vi "Peaks & Baseline.vi"(0 "Y data":dbl[](array[numeric]) format="%.2f", 1 "X interval (1.0)":dbl=1.0 format="%.2f", 2 "tuning parameters\n(0:auto-calc)":T1 {"peak threshold" min=0.0 format="%.2f"; "max noise" min=0.0 format="%.2f"}, 3 "iteration (0:init)":i32) -> (6 "baseline":T2 {"Y" format="%.2f"; "X" format="%.2f"}, 7 "X,Y data":T2 {"Y" format="%.2f"; "X" format="%.2f"}, 8 "peak starts":T2 {"Y" format="%.2f"; "X" format="%.2f"}, 9 "peak maxima":T2 {"Y" format="%.2f"; "X" format="%.2f"}, 10 "peak ends":T2 {"Y" format="%.2f"; "X" format="%.2f"})   [LabVIEW 2012]
doc: "The Peaks & Baseline VI finds the start, maximum, and end of each peak in a signal, and a linear baseline. This VI can process all the data at once (post-processing), or it can process the data in segments (\"on-line\" or \"real-time\" processing). It keeps state information from one call to the next by using uninitialized shift registers, so it can process segmented data seamlessly. Iteration must be set to zero for the first call so the state information can be initialized.\n\nUse the help window to read the descriptions of the individual controls for more information about this VI's inputs and outputs."
uses:
  XY Plot.ctl
  Tuning.ctl
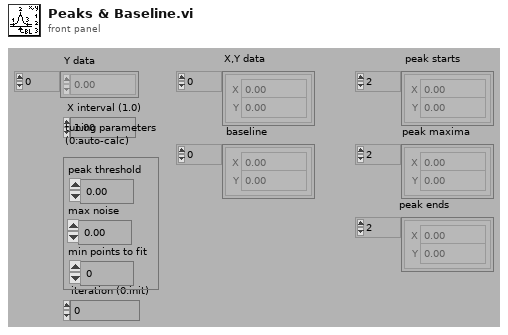
[diagram p1: front panel]
types:
  T1 = typedef "Tuning.ctl" = cluster{"max noise":dbl, "min points to fit":i32, "peak threshold":dbl}
  T2 = typedef "XY Plot.ctl" = cluster{"X":dbl, "Y":dbl}[]
  T3 = enum16{"initialize", "on baseline", "peak going up", "peak going down"}
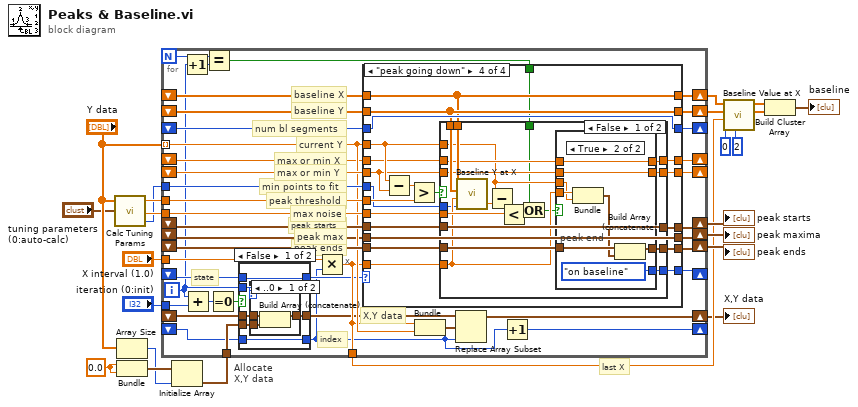
[diagram p0: block diagram]
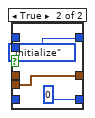
[diagram p3: hidden frame]
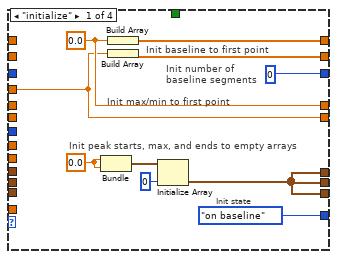
[diagram p4: hidden frame]
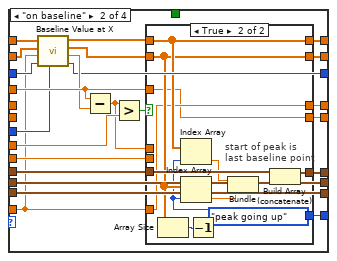
[diagram p5: hidden frame]
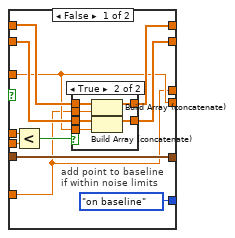
[diagram p6: hidden frame]
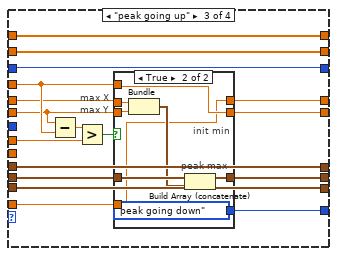
[diagram p8: hidden frame]
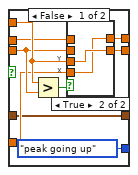
[diagram p9: hidden frame]
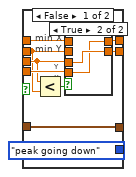
[diagram p11: hidden frame]
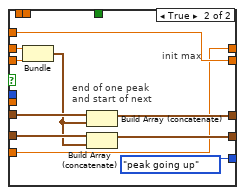
[diagram p13: hidden frame]
diagram:
  w11 = 0.0
  # "Allocate\nX,Y data"
  # "last X"
  n1 = call "Calc Tuning Params.vi"("tuning parameters\n(0:auto-calc)"="tuning parameters\n(0:auto-calc)", "Y data"="Y data") -> ("min points to fit"=w5:i32, "max noise"=w6:dbl, "peak threshold"=w7:dbl)  [unwired: 1 in]
  n2 = Array Size(array="Y data") -> (size(s)=w1:i32)
  n3 = Bundle(w11, w11) -> (w10:cluster{dbl, dbl})  [unwired: 1 in]
  n4 = Initialize Array(w10, w1) -> (w9:cluster{dbl, dbl}[])
  n5 = for {
    N -> [w25]
    shift-right: [w63] -> _
    shift-left: _ -> [w33]
    shift-right: [w55] -> _
    shift-left: _ -> [w56]
    tunnel: "Y data" -> [w47] mode=indexing
    shift-right: [w53] -> w19
    shift-left: _ -> [w62]
    shift-right: [w52] -> w18
    shift-left: _ -> [w61]
    shift-right: [w58] -> w16
    shift-left: _ -> [w60]
    shift-right: [w57] -> w14
    shift-left: _ -> [w59]
    tunnel: "X interval (1.0)" -> [w40]
    tunnel: w7 -> [w54]
    shift-right: [w51] -> _
    shift-left: _ -> [w50]
    tunnel: w5 -> [w49]
    tunnel: w6 -> [w48]
    shift-right: [w45] -> w12
    shift-left: _ -> [w34]
    shift-right: [w27] -> _
    shift-left: _ -> [w30]
    shift-right: [w43] -> _
    shift-left: _ -> [w44]
    shift-right: [w42] -> w15
    shift-left: _ -> [w41]
    tunnel: [w39] -> w13
    tunnel: w9 -> [w32]
    tunnel: "iteration (0:init)" -> [w29]
    i -> [w31]
    # "X,Y data"
    # "index"
    # "state"
    # "peak max"
    # "max or min X"
    # "max noise"
    # "min points to fit"
    # "peak threshold"
    # "num bl segments"
    # "max or min Y"
    # "peak starts"
    # "peak ends"
    # "baseline X"
    # "baseline Y"
    # "current Y"
    # "X"
    n6 = Increment(x=w31) -> (x+1=w24:i32)
    n7 = Add(x=w31, y=w29) -> (x+y=w36:i32)
    n8 = Equal?(x=w25, y=w24) -> (x = y?=w26:bool)
    n9 = Equal To 0?(x=w36) -> (x = 0?=w37:bool)
    n10 = case shown="False" w37 {
      tunnel: [w68 w75] -> w35
      tunnel: w34 -> [w69 _]
      tunnel: w33 -> [w67 _]
      tunnel: [w67 T3."initialize"] -> w38
      tunnel: w32 -> [w66 w75]
      tunnel: w31 -> [w65 _]
      tunnel: w30 -> [w64 _]
      tunnel: [w64 0] -> w28
      frame False {
        n11 = case shown="..0" w65 {
          tunnel: w69 -> [w72 w73]
          tunnel: w66 -> [w71 _]
          tunnel: [w70 w73] -> w68
          frame ..0 {
            n12 = Build Array (concatenate)(w72, w71) -> (w70:cluster{dbl, dbl}[])
          }
          frame 1.. {
          }
        }
      }
      frame True {
      }
    }
    n13 = Multiply(x=w40, y=w28) -> (x*y=w39:dbl)
    n14 = case shown="\"peak going down\"" w38 {
      tunnel: w47 -> [w77 w104 w146 w191]
      tunnel: w39 -> [_ w89 w141 w181]
      tunnel: [T3."on baseline" w107 w149 w193] -> w63
      tunnel: w62 -> [_ w100 w157 w187]
      tunnel: w61 -> [_ w99 w156 w188]
      tunnel: [w84 w109 w157 w187] -> w53
      tunnel: [w83 w108 w156 w188] -> w52
      tunnel: [w80 w103 w155 w195] -> w58
      tunnel: w60 -> [_ w102 w155 w196]
      tunnel: w59 -> [_ w101 w154 w197]
      tunnel: [w80 w101 w154 w194] -> w57
      tunnel: w54 -> [_ w105 w152 w186]
      tunnel: w56 -> [_ _ w145 w190]
      tunnel: [w77 w92 w150 w192] -> w55
      tunnel: [0 w87 w148 w189] -> w51
      tunnel: w50 -> [_ w98 w148 w189]
      tunnel: w49 -> [_ w95 _ w180]
      tunnel: w48 -> [_ w94 _ w185]
      tunnel: w44 -> [_ _ w144 w184]
      tunnel: [w81 w91 w147 w183] -> w43
      tunnel: [w80 w90 w142 w182] -> w42
      tunnel: w41 -> [_ w90 w143 w182]
      tunnel: w26 -> [_ _ _ w179]
      frame "initialize" {
        w81 = 0.0
        w86 = 0.0
        # "Init state"
        # "Init number of\nbaseline segments"
        # "Init max/min to first point"
        # "Init peak starts, max, and ends to empty arrays"
        # "Init baseline to first point"
        n15 = Bundle(w86, w86) -> (w78:cluster{dbl, dbl})  [unwired: 1 in]
        n16 = Build Array(w81) -> (w84:dbl[])
        n17 = Build Array(w77) -> (w83:dbl[])
        n18 = Initialize Array(w78, 0) -> (w80:cluster{dbl, dbl}[])
      }
      frame "on baseline" {
        n19 = call "Baseline Value at X.vi"("min points to fit (100)"=w95, "num segments before"=w98, "X"=w89, "baseline Y[]"=w99, "baseline X[]"=w100) -> ("num segments after"=w87:i32, "Y"=w96:dbl, "baseline Y[]"=w88:dbl[], "baseline X[]"=w97:dbl[])  [unwired: 1 in]
        n20 = Subtract(x=w104, y=w96) -> (x-y=w93:dbl)
        n21 = Greater?(x=w93, y=w105) -> (0:w106:bool)
        n22 = case shown="True" w106 {
          tunnel: w97 -> [w117 w139]
          tunnel: w89 -> [w110 w134]
          tunnel: w104 -> [w111 w129]
          tunnel: [w116 w139] -> w109
          tunnel: [w115 w138] -> w108
          tunnel: [T3."on baseline" T3."peak going up"] -> w107
          tunnel: w102 -> [w118 w140]
          tunnel: [w118 w136] -> w103
          tunnel: w94 -> [w113 _]
          tunnel: w93 -> [w112 _]
          tunnel: [w111 w129] -> w92
          tunnel: [w110 w134] -> w91
          tunnel: w88 -> [w120 w138]
          frame False {
            # "add point to baseline\nif within noise limits"
            n23 = Less?(x=w112, y=w113) -> (x < y?=w114:bool)
            n24 = case shown="True" w114 {
              tunnel: w117 -> [w122 w128]
              tunnel: [w122 w127] -> w116
              tunnel: [w121 w126] -> w115
              tunnel: w111 -> [_ w125]
              tunnel: w110 -> [_ w124]
              tunnel: w120 -> [w121 w123]
              frame False {
              }
              frame True {
                n25 = Build Array (concatenate)(w128, w124) -> (w127:dbl[])
                n26 = Build Array (concatenate)(w123, w125) -> (w126:dbl[])
              }
            }
          }
          frame True {
            # "start of peak is\nlast baseline point"
            n27 = Array Size(array=w138) -> (size(s)=w135:i32)
            n28 = Decrement(x=w135) -> (x-1=w133:i32)
            n29 = Index Array(array=w139, index=w133) -> (element=w131:dbl)
            n30 = Index Array(array=w138, index=w133) -> (element=w132:dbl)
            n31 = Bundle(w131, w132) -> (w130:cluster{dbl, dbl})  [unwired: 1 in]
            n32 = Build Array (concatenate)(w140, w130) -> (w136:cluster{dbl, dbl}[])
          }
        }
      }
      frame "peak going up" {
        # "max X"
        # "max Y"
        n33 = Subtract(x=w145, y=w146) -> (x-y=w153:dbl)
        n34 = Greater?(x=w153, y=w152) -> (0:w151:bool)
        n35 = case shown="True" w151 {
          tunnel: w146 -> [w165 w178]
          tunnel: w145 -> [w161 w173]
          tunnel: [w160 w178] -> w150
          tunnel: [T3."peak going up" T3."peak going down"] -> w149
          tunnel: w141 -> [w159 w171]
          tunnel: [w162 w171] -> w147
          tunnel: w144 -> [w163 w174]
          tunnel: w143 -> [w158 w176]
          tunnel: [w158 w175] -> w142
          frame False {
            # "X"
            # "Y"
            n36 = Greater?(x=w165, y=w161) -> (0:w164:bool)
            n37 = case shown="True" w164 {
              tunnel: [w167 w170] -> w160
              tunnel: [w168 w169] -> w162
              tunnel: w163 -> [w168 _]
              tunnel: w165 -> [_ w170]
              tunnel: w161 -> [w167 _]
              tunnel: w159 -> [_ w169]
              frame False {
              }
              frame True {
              }
            }
          }
          frame True {
            # "peak max"
            # "init min"
            n38 = Bundle(w174, w173) -> (w172:cluster{dbl, dbl})  [unwired: 1 in]
            n39 = Build Array (concatenate)(w176, w172) -> (w175:cluster{dbl, dbl}[])
          }
        }
      }
      frame "peak going down" {
        n40 = Subtract(x=w191, y=w190) -> (x-y=w199:dbl)
        n41 = Greater?(x=w199, y=w186) -> (0:w198:bool)
        n42 = case shown="False" w198 {
          tunnel: [w217 T3."peak going up"] -> w193
          tunnel: w181 -> [w204 w243]
          tunnel: [w212 w249] -> w195
          tunnel: w191 -> [w207 w244]
          tunnel: w197 -> [w211 w248]
          tunnel: w196 -> [w212 w247]
          tunnel: [w210 w246] -> w194
          tunnel: [w205 w244] -> w192
          tunnel: w185 -> [w215 _]
          tunnel: w190 -> [w208 w241]
          tunnel: w188 -> [w218 _]
          tunnel: w187 -> [w213 _]
          tunnel: w184 -> [w209 w242]
          tunnel: [w206 w243] -> w183
          tunnel: w180 -> [w203 _]
          tunnel: w179 -> [w200 _]
          frame False {
            n43 = call "Baseline Y at X.vi"("min points to fit (100)"=w203, "X"=w204, "baseline Y[]"=w218, "baseline X[]"=w213) -> ("Y"=w214:dbl)  [unwired: 1 in]
            n44 = Subtract(x=w207, y=w214) -> (x-y=w216:dbl)
            n45 = Less?(x=w216, y=w215) -> (x < y?=w202:bool)
            n46 = Or(x=w200, y=w202) -> (x .or. y?=w201:bool)
            n47 = case shown="True" w201 {
              tunnel: [T3."peak going down" T3."on baseline"] -> w217
              tunnel: w211 -> [w226 w238]
              tunnel: [w226 w237] -> w210
              tunnel: w209 -> [w225 w236]
              tunnel: w208 -> [w220 w235]
              tunnel: w207 -> [w221 w233]
              tunnel: w204 -> [w224 w234]
              tunnel: [w223 w236] -> w206
              tunnel: [w222 w235] -> w205
              frame False {
                # "min X"
                # "min Y"
                # "Y"
                # "X"
                n48 = Less?(x=w221, y=w220) -> (x < y?=w219:bool)
                n49 = case shown="True" w219 {
                  tunnel: [w229 w231] -> w222
                  tunnel: w220 -> [w229 _]
                  tunnel: [w228 w230] -> w223
                  tunnel: w225 -> [w228 _]
                  tunnel: w224 -> [_ w230]
                  tunnel: w221 -> [_ w231]
                  frame False {
                  }
                  frame True {
                  }
                }
              }
              frame True {
                # "peak end"
                n50 = Bundle(w234, w233) -> (w232:cluster{dbl, dbl})  [unwired: 1 in]
                n51 = Build Array (concatenate)(w238, w232) -> (w237:cluster{dbl, dbl}[])
              }
            }
          }
          frame True {
            # "init max"
            # "end of one peak\nand start of next"
            n52 = Bundle(w242, w241) -> (w240:cluster{dbl, dbl})  [unwired: 1 in]
            n53 = Build Array (concatenate)(w247, w240) -> (w249:cluster{dbl, dbl}[])
            n54 = Build Array (concatenate)(w248, w240) -> (w246:cluster{dbl, dbl}[])
          }
        }
      }
    }
    n55 = Bundle(w39, w47) -> (w46:cluster{dbl, dbl})  [unwired: 1 in]
    n56 = Replace Array Subset(array=w35, new element=w46, index=w28) -> (w45:cluster{dbl, dbl}[])
    n57 = Increment(x=w28) -> (x+1=w27:i32)
  }
  "X,Y data" <- w12
  "peak ends" <- w14
  "peak maxima" <- w15
  "peak starts" <- w16
  n58 = call "Baseline Value at X.vi"("min points to fit (100)"=2, "num segments before"=0, "X"=w13, "baseline Y[]"=w18, "baseline X[]"=w19) -> ("baseline Y[]"=w20:dbl[], "baseline X[]"=w21:dbl[])  [unwired: 1 in, 2 out]
  n59 = Build Cluster Array(w21, w20) -> (→"baseline":cluster{dbl, dbl}[])
